vi "Read Lab Spectrum.VI"(6 "Aktionen":T3, 8 "error in (no error)":errorcluster caption="Fehler (Eingang, kein Fehler)", 9 "Auswahl":T2, 11 "Spectrum  FILE Name":path=path "C:/OLT/backgrnd.lab") -> (0 "error out":errorcluster caption="Fehler (Ausgang)", 1 "Graph 1":T1, 2 "Graph":cluster{dbl[], sgl[]}, 3 "Zeitstempel":timestamp)   [LabVIEW 2020, in "FT-IR.lvlib" / "Read Lab File.lvlib"]
uses:
  Read Lab File.lvlib
  Aktionen Lab File.ctl
  Aswahl Lab File.ctl
  Grafik/Diagramm_NEU.ctl
  Spectrum FILE.ctl
  User arrays.ctl
  Sub spectra.ctl
  Spectrum.ctl
  Grafik/Grafik.lvlib
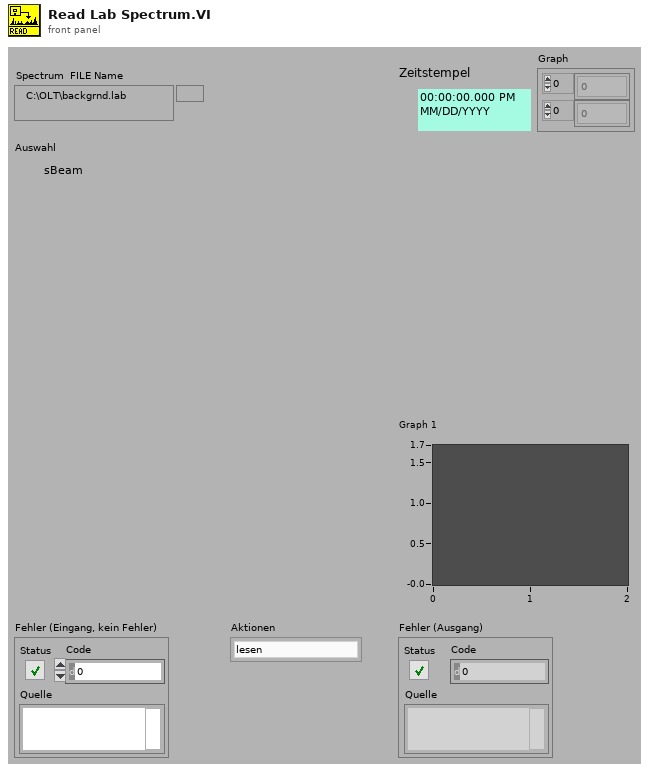
[diagram p1: front panel]
types:
  T1 = typedef "Grafik.lvlib/Diagramm_NEU.ctl" = waveform(dbl)
  T2 = typedef "FT-IR.lvlib/Read Lab File.lvlib/Aswahl Lab File.ctl" = enum16{"sBeam", "Main", "igram", "Previous"}
  T3 = typedef "FT-IR.lvlib/Read Lab File.lvlib/Aktionen Lab File.ctl" = enum16{"lesen", "laden"}
  T4 = typedef "FT-IR.lvlib/Read Lab File.lvlib/Spectrum FILE.ctl" = cluster{"MEMO":string, "User arrays":T5, "SPECTRA":T6}
  T5 = typedef "FT-IR.lvlib/Read Lab File.lvlib/User arrays.ctl" = cluster{"Tag":string, "User double":dbl[]}[]
  T6 = typedef "FT-IR.lvlib/Read Lab File.lvlib/Sub spectra.ctl" = cluster{"Tag":string, "DATE AND TIME":u32, "spectrum":T7}[]
  T7 = typedef "FT-IR.lvlib/Read Lab File.lvlib/Spectrum.ctl" = cluster{"x0":dbl, "dx":dbl, "[Y]":sgl[]}
  T8 = cluster{"Tag":string, "DATE AND TIME":u32, "spectrum":T7}
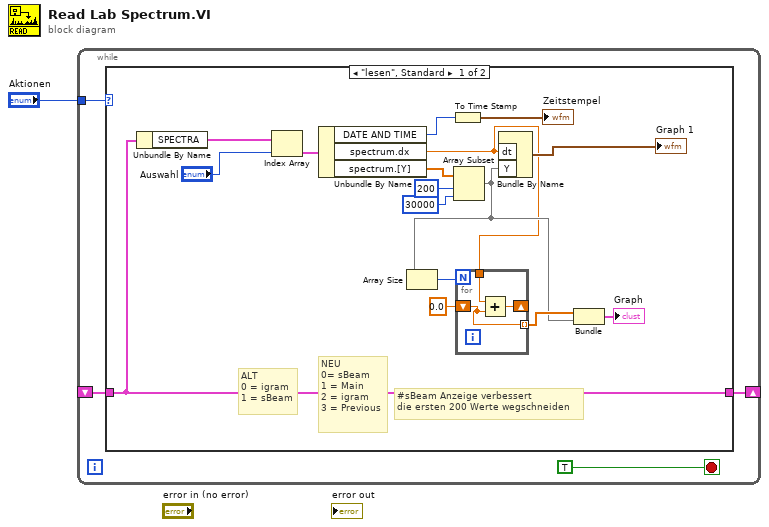
[diagram p0: block diagram]
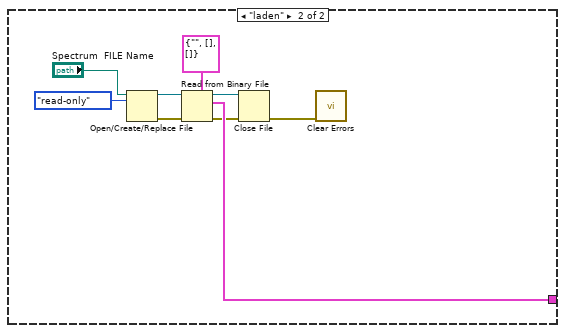
[diagram p2: hidden frame]
diagram:
  n1 = while {
    shift-right: [w5] -> _
    shift-left: _ -> [w4]
    tunnel: "Aktionen" -> [w3]
    stop <- TRUE stop-if-true
    n2 = case shown="\"lesen\", Standard" w3 {
      tunnel: [w18 w30] -> w5
      tunnel: w4 -> [w18 _]
      frame "lesen", Default {
        # "#sBeam Anzeige verbessert\ndie ersten 200 Werte wegschneiden"
        # "NEU\n0= sBeam\n1 = Main\n2 = igram\n3 = Previous"
        # "ALT\n0 = igram\n1 = sBeam"
        n3 = Unbundle By Name(w18) -> ("SPECTRA"=w19:T6)
        n4 = Index Array(array=w19, index="Auswahl") -> (element=w20:T8)
        n5 = Unbundle By Name(w20) -> ("DATE AND TIME"=w21:u32, "spectrum.dx"=w7:dbl, "spectrum.[Y]"=w13:sgl[])
        n6 = To Time Stamp(1:w21) -> (0:→"Zeitstempel":timestamp)
        n7 = Array Subset(array=w13, index=200 ("Index"), length=30000 ("Länge")) -> (w8:sgl[])
        n8 = Array Size(array=w8) -> (size(s)=w10:i32)
        n9 = for {
          N: w10 -> [_]
          tunnel: [w23] -> w11 mode=indexing
          shift-right: [w24] -> _
          shift-left: 0.0 -> [w23]
          tunnel: w7 -> [w22]
          n10 = Add(x=w22, y=w23) -> (x+y=w24:dbl)
        }
        n11 = Bundle By Name("dt"=w7, "Y"=w8) -> (→"Graph 1":waveform(sgl))  [unwired: 1 out]
        n12 = Bundle(w11, w8) -> (→"Graph":cluster{dbl[], sgl[]})  [unwired: 1 in]
      }
      frame "laden" {
        n13 = Open/Create/Replace File(file path (use dialog)="Spectrum  FILE Name", access (0:read/write)=enum16{"read/write", "read-only", "write-only"}."read-only" ("Zugriff (0:Lesen/Schreiben)")) -> (refnum out=w33:refnum<file>, error out=w32:errorcluster)  [unwired: 1 in, 4 out]
        n14 = Read from Binary File(5:T4 {"MEMO"="", "User arrays"=[], "SPECTRA"=[]} ("empty Spectrum FILE"), 8:w32, 11:w33) -> (0:w27:errorcluster, 2:w30:T4, 3:w31:refnum<file>)  [unwired: 4 out]
        n15 = Close File(refnum=w31, error in=w27) -> (error out=w25:errorcluster)  [unwired: 1 out]
        n16 = call <vilib>:"Clear Errors.vi"("error in (no error)"=w25) -> ()  [unwired: 5 in, 2 out]
      }
    }
  }
